vi "IR_Alignment_Diode.vi"(0 "AD Action":enum16{"AD Off", "AD On"}(ring)) -> (15 "error_Code":i32)   [LabVIEW 2015]
uses:
  OPOTEK.dll
panel:
  # "AD Control"
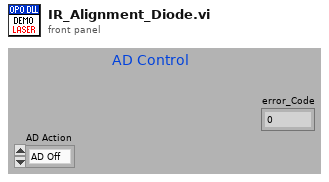
[diagram p1: front panel]
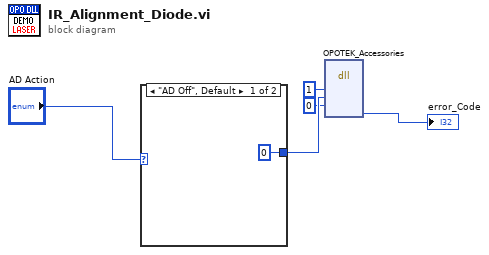
[diagram p0: block diagram]
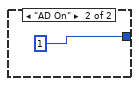
[diagram p2: hidden frame]
diagram:
  n1 = case shown="\"AD Off\", Default" "AD Action" {
    tunnel: [0 1] -> w3
    frame "AD Off", Default {
    }
    frame "AD On" {
    }
  }
  n2 = dll-call lib="C:/Users/SuperMicro/Desktop/LabView/IR Opolette Controller/OPOTEK.dll" fn="OPOTEK_Accessories"("action"=i8 1, "parameter1"=w3, "parameter2"=i16 0) -> ("error_Code"=→"error_Code":i32)  [unwired: 8 in, 2 out]
